vi "initialize vi references.vi"(8 "error in":errorcluster, 9 "config class path":path, 10 "runtime class path":path, 11 "spec":T1[](array[typedef])) -> (0 "error out":errorcluster, 3 "initialized references":T3[](array[typedef]))   [LabVIEW 2013, in "control module data interface generator.lvlib"]
uses:
  control module data interface generator.lvlib
  Controls/initialized references.ctl
  Controls/interface VI type.ctl
  Controls/scripting spec.ctl
  <vilib>/NI/Tag Bus Module Framework/channel/channel classification.ctl
  <vilib>/NI/Tag Bus Module Framework/channel/TBM channel.lvclass
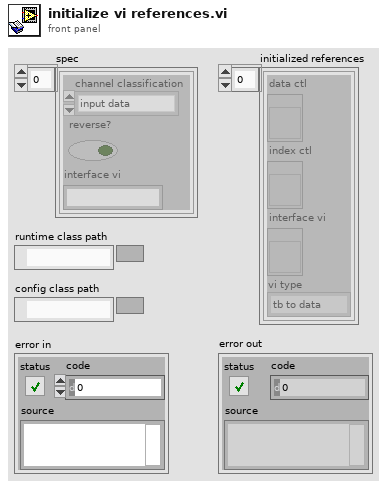
[diagram p1: front panel]
types:
  T1 = typedef "control module data interface generator.lvlib/scripting spec.ctl" = cluster{"channel classification":T2, "reverse?":bool, "interface vi":string}
  T2 = typedef "TBM channel.lvclass/channel classification.ctl" = enum16{"input data", "output data", "processing parameter", "processing result"}
  T3 = typedef "control module data interface generator.lvlib/initialized references.ctl" = cluster{"data ctl":refnum<vi>, "index ctl":refnum<vi>, "interface vi":refnum<vi>, "vi type":T4}
  T4 = typedef "control module data interface generator.lvlib/interface VI type.ctl" = enum16{"tb to data", "data to tb"}
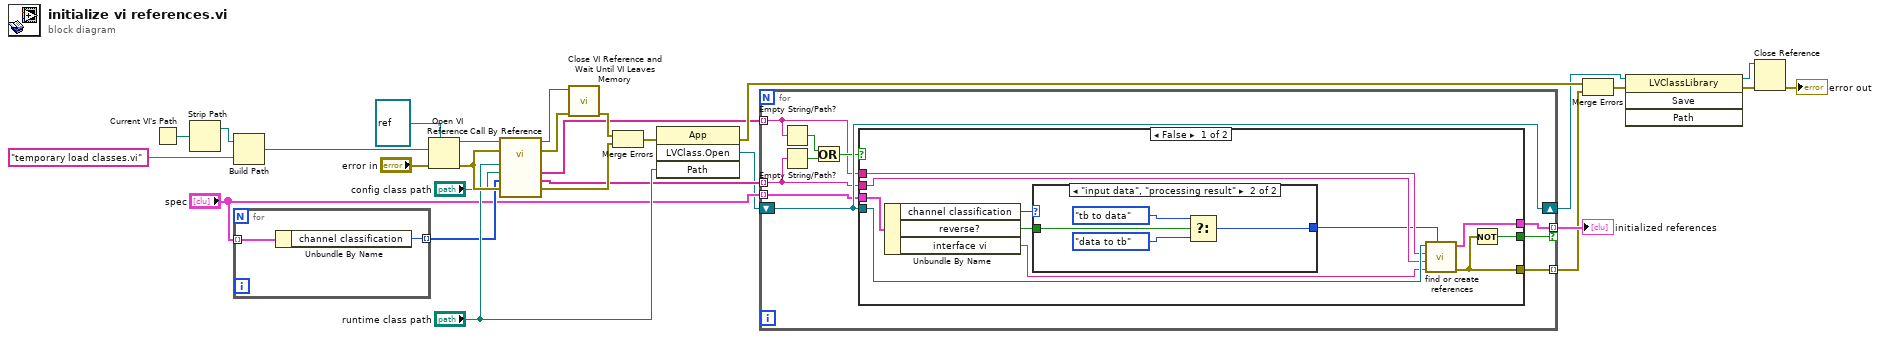
[diagram p0: block diagram]
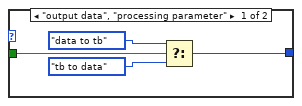
[diagram p2: hidden frame]
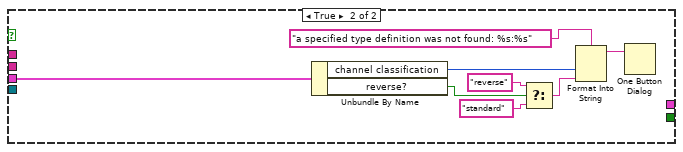
[diagram p3: hidden frame]
diagram:
  n1 = Current VI's Path() -> (path=w23:path)
  n2 = Strip Path(path=w23) -> (stripped path=w22:path)  [unwired: 1 out]
  n3 = Build Path(base path=w22, name or relative path="temporary load classes.vi") -> (appended path=w20:path)
  n4 = for {
    tunnel: "spec" -> [w30] mode=indexing
    tunnel: [w29] -> w8 mode=indexing
    n5 = Unbundle By Name(w30) -> ("channel classification"=w29:T2)
  }
  n6 = Open VI Reference(type specifier VI Refnum (for type only)=refnum<vi> refnum, vi path=w20, error in (no error)="error in") -> (vi reference=w18:refnum<vi>, error out=w13:errorcluster)  [unwired: 3 in]
  n7 = call-by-ref "?"(reference=w18, error in=w13, "error in"=w13, "classifications"=w8, "config class path"="config class path", "runtime class path"="runtime class path") -> (reference out=w16:refnum<vi>, error out=w17:errorcluster, 0:"error out"=w11:errorcluster, "index ctl"=w5:string[], "data ctl"=w6:string[])  [unwired: 4 in, 1 out]
  n8 = call <vilib>:"Close VI Reference and Wait Until VI Leaves Memory.vi"("error in (no error)"=w17, "VI reference"=w16) -> ("error out"=w15:errorcluster)  [unwired: 9 in]
  n9 = Merge Errors(w15, w11) -> (w12:errorcluster)
  n10 = invoke class="App" method="LVClass.Open"(error in=w12, "Path"="runtime class path") -> (error out=w27:errorcluster, "LVClass.Open"=w4:refnum<vi>)  [unwired: 2 in, 2 out]
  n11 = for {
    tunnel: "spec" -> [w34] mode=indexing
    tunnel: w6 -> [w33] mode=indexing
    tunnel: w5 -> [w32] mode=indexing
    shift-right: [w40] -> w3
    shift-left: w4 -> [w40]
    tunnel: [w39] -> w2 mode=indexing if=w38
    tunnel: [w31] -> w1 mode=indexing
    n12 = Empty String/Path?(string/path=w33) -> (empty?=w36:bool)
    n13 = Empty String/Path?(string/path=w32) -> (empty?=w37:bool)
    n14 = Or(x=w36, y=w37) -> (x .or. y?=w35:bool)
    n15 = case shown="False" w35 {
      tunnel: w40 -> [w51 _]
      tunnel: [w50 _] -> w39
      tunnel: [w49 _] -> w38
      tunnel: w34 -> [w48 w67]
      tunnel: w33 -> [w46 _]
      tunnel: w32 -> [w45 _]
      tunnel: [w41 _] -> w31
      frame False {
        n16 = Unbundle By Name(w48) -> ("channel classification"=w44:T2, "reverse?"=w43:bool, "interface vi"=w47:string)
        n17 = case shown="\"input data\", \"processing result\"" w44 {
          tunnel: w43 -> [w55 w59]
          tunnel: [w52 w56] -> w42
          frame "output data", "processing parameter" {
            n18 = Select(t=interface_VI_type."data to tb" ("vi type"), s=w55, f=interface_VI_type."tb to data" ("vi type")) -> (s? t:f=w52:T4)
          }
          frame "input data", "processing result" {
            n19 = Select(t=interface_VI_type."tb to data" ("vi type"), s=w59, f=interface_VI_type."data to tb" ("vi type")) -> (s? t:f=w56:T4)
          }
        }
        n20 = call "find or create references.vi"("vi type"=w42, "Data Interface VI"=w47, "index ctl"=w45, "data ctl"=w46, "runtime"=w51) -> ("error out"=w41:errorcluster, "vi refs"=w50:T3)  [unwired: 5 in]
        n21 = Not(x=w41) -> (.not. x?=w49:bool)
      }
      frame True {
        n22 = Unbundle By Name(w67) -> ("channel classification"=w61:T2, "reverse?"=w65:bool)
        n23 = Select(t="reverse", s=w65, f="standard") -> (s? t:f=w62:string)
        n24 = Format Into String(format string="a specified type definition was not found: %s:%s", w61, w62) -> (resulting string=w60:string)  [unwired: 2 in, 1 out]
        n25 = One Button Dialog(message=w60) -> ()  [unwired: 1 in, 1 out]
      }
    }
  }
  "initialized references" <- w2
  n26 = Merge Errors(w27, w1) -> (w28:errorcluster)
  n27 = invoke class="LVClassLibrary" method="Save"(reference=w3, error in=w28) -> (reference out=w25:refnum<vi>, error out=w26:errorcluster)  [unwired: 2 in, 2 out]
  n28 = Close Reference(reference=w25, error in (no error)=w26) -> (error out=→"error out":errorcluster)
